vi "CH_LM Action Position Stability Cycle StartStop.vi"(0 "Meter Index":i32, 2 "Start/Stop (start)":bool=TRUE, 5 "error in (no error)":errorcluster, 7 "Timeout / ms (3000)":i32=3000, 9 "Lock Timeout / ms (1000)":i32=1000) -> (11 "Lock timed out":bool, 14 "Meter Index":i32, 19 "error out":errorcluster)   [LabVIEW 2012, in "CH_LM.lvlib"]
doc: "This command will initiate/restart or terminate a position stability display cycle.\n\n</B>Note:</B> This command will be ignored if a position stability display mode is not active or a position stability display cycle is not in progress."
uses:
  CH_LM.lvlib
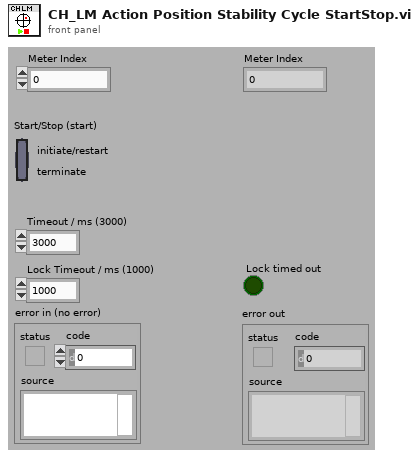
[diagram p1: front panel]
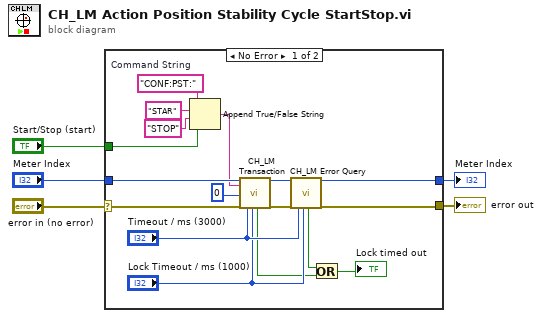
[diagram p0: block diagram]
diagram:
  n1 = case shown="No Error" "error in (no error)" {
    selector: "error in (no error)" -> [w22 w24]
    tunnel: [w20 w24] -> w5
    tunnel: "Meter Index" -> [w21 w23]
    tunnel: [w19 w23] -> w2
    tunnel: "Start/Stop (start)" -> [w8 _]
    frame No Error {
      w11 = "CONF:PST:"  # Command String
      n2 = Append True/False String(1:w8, 2:"STOP" ("false string"), 3:"STAR" ("true string"), 4:w11) -> (0:w10:string)
      n3 = call "CH_LM Transaction.vi"("Meter Index"=w21, "Command String"=w10, "NofStrings (-1:all)"=0 ("t"), "error in (no error)"=w22, "Timeout / ms (3000)"="Timeout / ms (3000)", "Lock Timeout / ms (1000)"="Lock Timeout / ms (1000)") -> ("Lock timed out"=w13:bool, "Meter Index"=w16:i32, "error out"=w15:errorcluster)  [unwired: 11 out]
      n4 = call "CH_LM Error Query.vi"("Meter Index"=w16, "error in (no error)"=w15, "Timeout / ms (3000)"="Timeout / ms (3000)", "Lock Timeout / ms (1000)"="Lock Timeout / ms (1000)") -> ("Lock timed out"=w14:bool, "Meter Index"=w19:i32, "error out"=w20:errorcluster)  [unwired: 13 out]
      n5 = Or(x=w14, y=w13) -> (x .or. y?=→"Lock timed out":bool)
    }
    frame Error {
    }
  }
  "error out" <- w5
  "Meter Index" <- w2
